vi "PSDATA_Variant To AWFM.vi"(9 "error in":errorcluster, 10 "Value":variant) -> (1 "error out":errorcluster, 2 "Value":string, 4 "AWFM":waveform(dbl)(graph))   [LabVIEW 2016]
doc: "Developer：YDX"
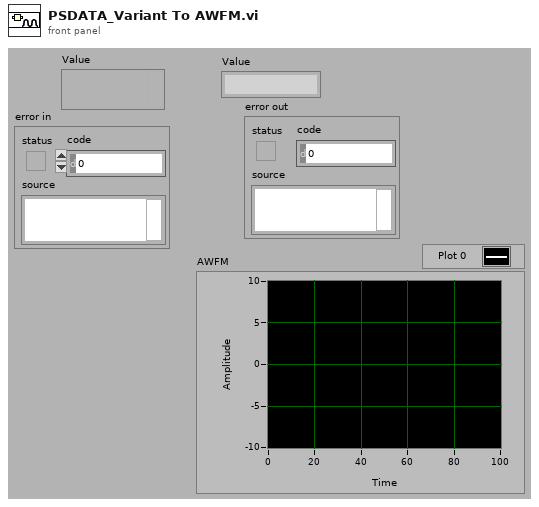
[diagram p1: front panel]
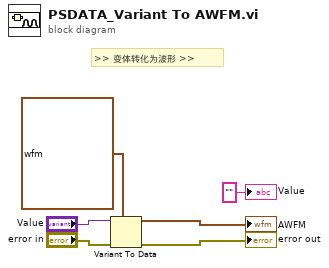
[diagram p0: block diagram]
diagram:
  # ">> 变体转化为波形 >>"
  n1 = Variant To Data(error in="error in", type=waveform(dbl) {"t0"=timestamp(0 s since 1904-01-01), "dt"=1.0, "Y"=[]} ("waveform"), Variant="Value") -> (data=→"AWFM":waveform(dbl), error out=→"error out":errorcluster)
  "Value" <- "" ("Value")
